vi "set out plane position.vi"(9 "Speed":dbl=1.0 format="%#_13g", 10 "Instrument":T1 {"Input (1;B)" items=["A", "B"]; "Input (0:A) 325" items=["A", "B"]; "Input (0:A)" items=["A", "B"]; "Heater Output (1:1)" items=["1"=1, "2"=2]}, 11 "Value":dbl) -> ()   [LabVIEW 2019, in "9T cmag.lvlib"]
uses:
  9T cmag.lvlib
  ctl/Instrument.ctl
  <vilib>/NI/Modbus Library/API/Master/Modbus Master.lvclass
  ctl/Instrument Type.ctl
  lib/QDInstrument.dll
  ctl/335 state.ctl
  ctl/limit.ctl
  ctl/9T mag field stauts.ctl
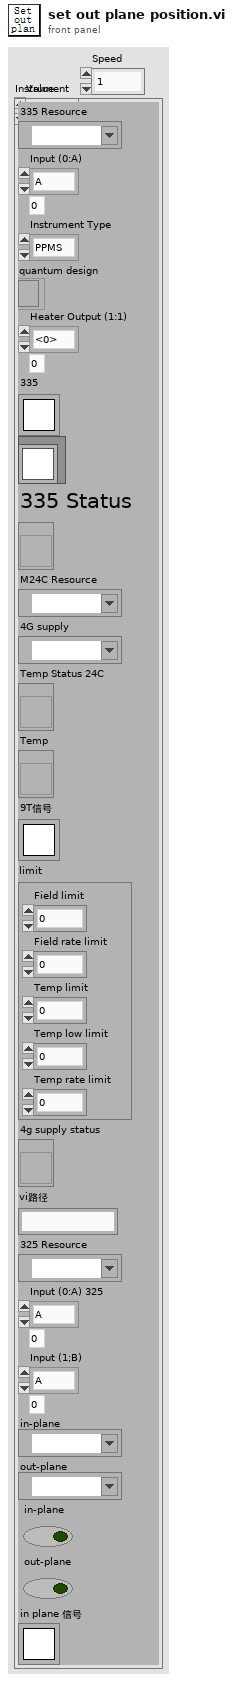
[diagram p1: front panel]
types:
  T1 = typedef "Instrument.ctl" = cluster{"335 Resource":refnum<visa-resource-name>, "Input (0:A)":u16, "Instrument Type":T2, "quantum design":refnum<k24>, "Heater Output (1:1)":u16, "semaphore":T3, "TCP master instance":refnum<class "Modbus Master.lvclass">, "335 Status":refnum<vi>, "M24C Resource":refnum<visa-resource-name>, "4G supply":refnum<visa-resource-name>, "Temp Status 24C":refnum<vi>, "Temp":refnum<vi>, "9T信号":T3, "limit":T4, "4g supply status":refnum<vi>, "vi路径":string, "325 Resource ":refnum<visa-resource-name>, "Input (0:A) 325":u16, "Input (1;B)":u16, "in-plane":refnum<visa-resource-name>, "out-plane":refnum<visa-resource-name>, "in-plane":bool, "out-plane":bool, "in plane 信号":T3}
  T2 = typedef "Instrument Type.ctl" = enum16{"PPMS", "VersaLab", "DynaCool", "SVSM", "PPMS-Rotate", "Lakeshore335", "9T mag"}
  T3 = typedef "Semaphore RefNum" = refnum<k1>
  T4 = typedef "limit.ctl" = cluster{"Field limit":dbl, "Field rate limit":dbl, "Temp limit":dbl, "Temp low limit":dbl, "Temp rate limit ":dbl}
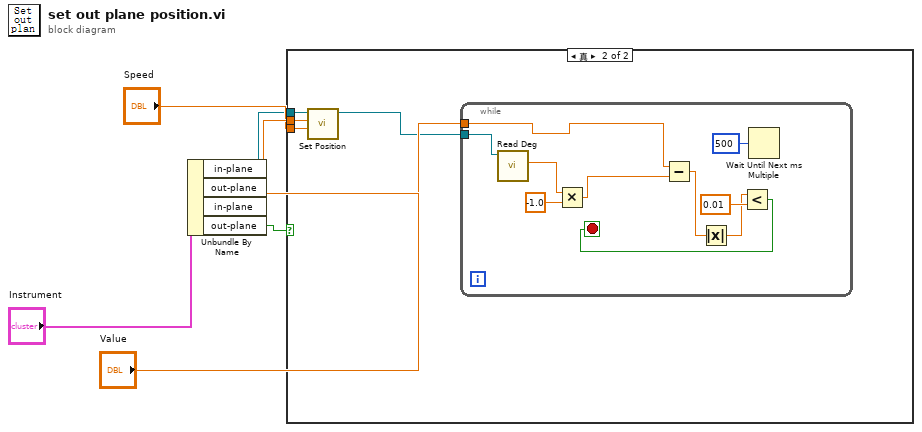
[diagram p0: block diagram]
diagram:
  n1 = Unbundle By Name("Instrument") -> ("out-plane"=w3:refnum<visa-resource-name>, "out-plane"=w1:bool)  [unwired: 2 out]
  n2 = case shown="真" w1 {
    tunnel: "Value" -> [_ w9]
    tunnel: "Speed" -> [_ w7]
    tunnel: w3 -> [_ w6]
    frame False {
    }
    frame True {
      n3 = call "Set Position.vi"("Speed"=w7, "Target"=w9, "VISA resource name in"=w6) -> ("VISA resource name out"=w8:refnum<visa-resource-name>)  [unwired: 7 in, 1 out]
      n4 = while {
        tunnel: w8 -> [w19]
        tunnel: w9 -> [w15]
        stop <- w11 stop-if-true
        n5 = call "Read Deg.vi"("VISA resource name out"=w19) -> ("角度"=w18:dbl)  [unwired: 8 in, 2 out]
        n6 = Multiply(x=w18, y=-1.0) -> (x*y=w14:dbl)
        n7 = Subtract(x=w15, y=w14) -> (x-y=w12:dbl)
        n8 = Absolute Value(x=w12) -> (abs(x)=w10:dbl)
        n9 = Less?(x=w10, y=0.01) -> (x < y?=w11:bool)
        n10 = Wait Until Next ms Multiple(millisecond multiple=u32 500 ("毫秒倍数")) -> ()  [unwired: 1 out]
      }
    }
  }
